vi "CreateCore.vi"(8 "error in (no error)":errorcluster, 10 "ParamsArray":variant[](array[variant]), 11 "ConcreteProductA in":refnum<class "ConcreteProductB.lvclass">) -> (0 "error out":errorcluster, 3 "ConcreteProductA out":refnum<class "ConcreteProductB.lvclass">)   [LabVIEW 2020, in "FactoryMethod.lvlib" / "ConcreteProductB.lvclass"]
uses:
  ConcreteProductB.lvclass
  ConcreteProductB.lvclass/ConcreteProductB.ctl
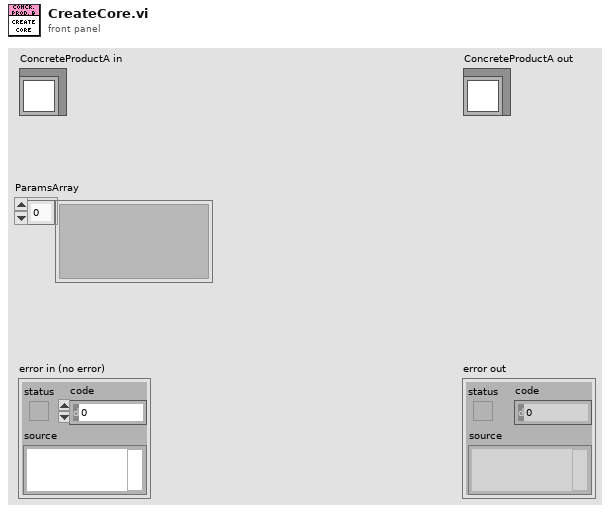
[diagram p1: front panel]
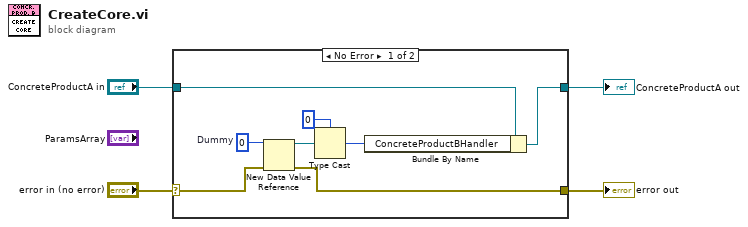
[diagram p0: block diagram]
diagram:
  n1 = case shown="No Error" "error in (no error)" {
    selector: "error in (no error)" -> [w6 w14]
    tunnel: [w7 w14] -> w1
    tunnel: [w9 w13] -> w3
    tunnel: "ConcreteProductA in" -> [w8 w13]
    frame No Error {
      w5 = u8 0  # Dummy
      n2 = New Data Value Reference(data value=w5, error in=w6) -> (data value reference=w12:refnum<data-value>, error out=w7:errorcluster)
      n3 = Type Cast(type=u32 0, x=w12) -> (*(type *) &x=w10:u32)
      n4 = Bundle By Name(cluster=w8, "ConcreteProductBHandler"=w10) -> (w9:refnum<class "ConcreteProductB.lvclass">)
    }
    frame Error {
    }
  }
  "error out" <- w1
  "ConcreteProductA out" <- w3
